vi "ErrorCheck.vi"(0 "Calib Baud rate":u32=9600, 1 "External VRN (COM8)":refnum<visa-resource-name>="COM8", 2 "Input Baud rate":u32=38400, 3 "TCS C VRN (COM4)":refnum<visa-resource-name>="COM4", 4 "TCS Contrôle Baud rate":u32=57600, 5 "TCS R VRN (COM7)":refnum<visa-resource-name>="COM7", 6 "TCS Requête Baud rate":u32=57600, 7 "MC bonOMM (COM3)":refnum<visa-resource-name>="COM3", 8 "Calib VRN (COM5)":refnum<visa-resource-name>="COM5", 9 "PathArray":path[](array[path])=[path "C:/UdeM/BonOMM-10/BonOMM-10_nocmd.vi", path "C:/UdeM/BonOMM-10/tracklogfiles", path "C:/UdeM/BonOMM-10/systemlogfiles", path "C:/UdeM/BonOMM-10/objectlibrary"], 10 "Table Baud rate":u32=38400, 12 "Table VRN (COM9)":refnum<visa-resource-name>="COM9") -> (11 "sortie librarypath":path=path "C:/UdeM/BonOMM-10/objectlibrary", 13 "sortie track":path=path "C:/UdeM/BonOMM-10/tracklogfiles", 14 "Table VRN OUT":refnum<visa-resource-name>="-1", 15 "sortie systemlog":path=path "C:/UdeM/BonOMM-10/systemlogfiles", 16 "Table Baud rate":u32=38400, 17 "Initialistion ok!":bool=TRUE, 18 "Calib VRN OUT":refnum<visa-resource-name>="COM5", 19 "MODE ?":i16=4, 20 "Calib Baud rate 2":u32=9600, 21 "External VRN OUT":refnum<visa-resource-name>="COM8", 22 "Input Baud rate 2":u32=38400, 23 "TCS C VRN OUT":refnum<visa-resource-name>="-1", 24 "TCS Contrôle Baud rate 2":u32=57600, 25 "TCS R VRN OUT":refnum<visa-resource-name>="-1", 26 "TCS Requête Baud rate":u32=57600, 27 "MC bonOMM OUT":refnum<visa-resource-name>="COM3")   [LabVIEW 2010]
uses:
  Comm/InitSerialPort_option.vi
panel:
  in  "search_MCB":bool
  in  "objectlibrarypath":path=path "C:/UdeM/BonOMM-10/objectlibrary" caption="Chemin du dossier des librairies"
  out "progress":i32(slide) min=0 max=100 step=5 scale=0.0..100.0
  out "MC Baud rate 2":u32=9600
  out "sortie vipath":path=path "C:/UdeM/BonOMM-10/BonOMM-10_nocmd.vi"
  in  "systemlogfilepath":path=path "C:/UdeM/BonOMM-10/systemlogfiles"
  in  "trackfilepath":path=path "C:/UdeM/BonOMM-10/tracklogfiles"
  in  "vipath":path=path "C:/UdeM/BonOMM-10/BonOMM-10_nocmd.vi"
  out "SPECTRO VRN OUT":refnum<visa-resource-name>="COM7"
  out "SPECTRO Baud rate":u32=57600
  out "ok 6":bool
  in  "MC Baud rate":u32=9600
  out "ok 5":bool
  out "ok 4":bool
  out "ok 3":bool
  out "ok 2":bool
  out "ok 1":bool
  in  "Annuler":bool
  in  "Démarrer":bool
  # "Chemin de l'application"
  # "Chemin des trackfiles"
  # "Chemin du dossier des logs système"
  # "Appuyer sur DÉMARRER lorsque vous\nêtes prêt à éxécuter BonOMM"
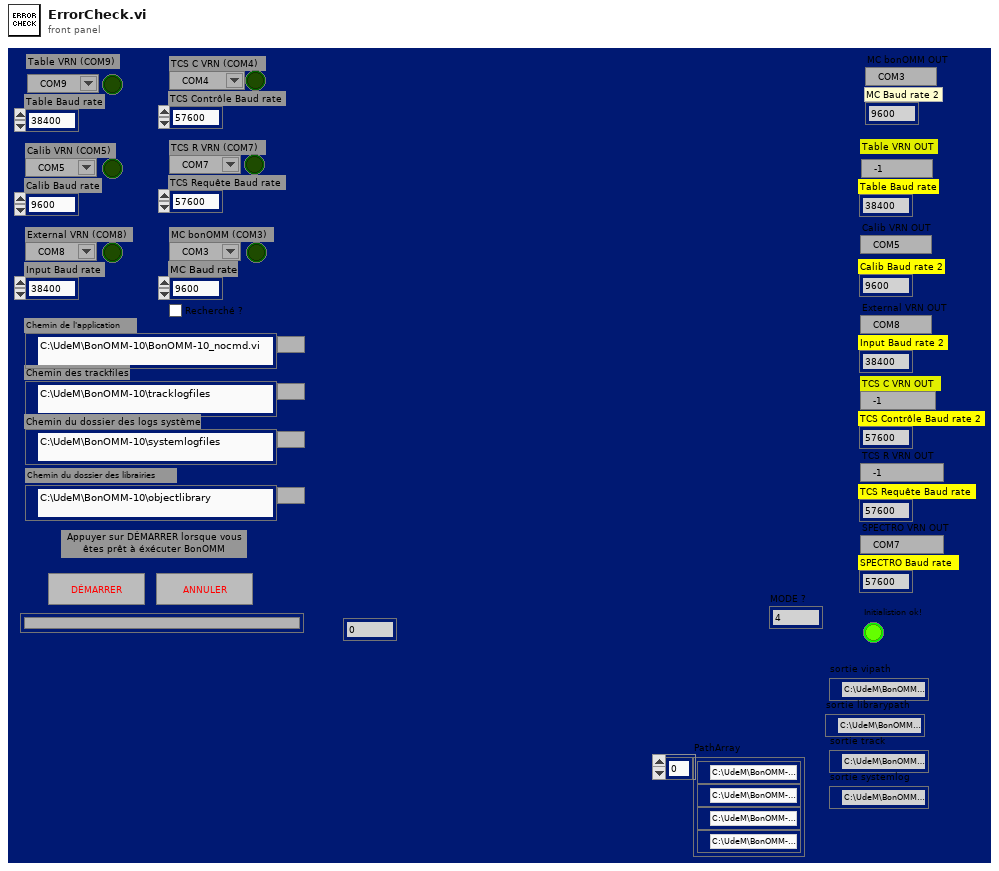
[diagram p1: front panel]
types:
  T1 = enum16{"Left Button", "Center Button", "Right Button", "Window Close"}
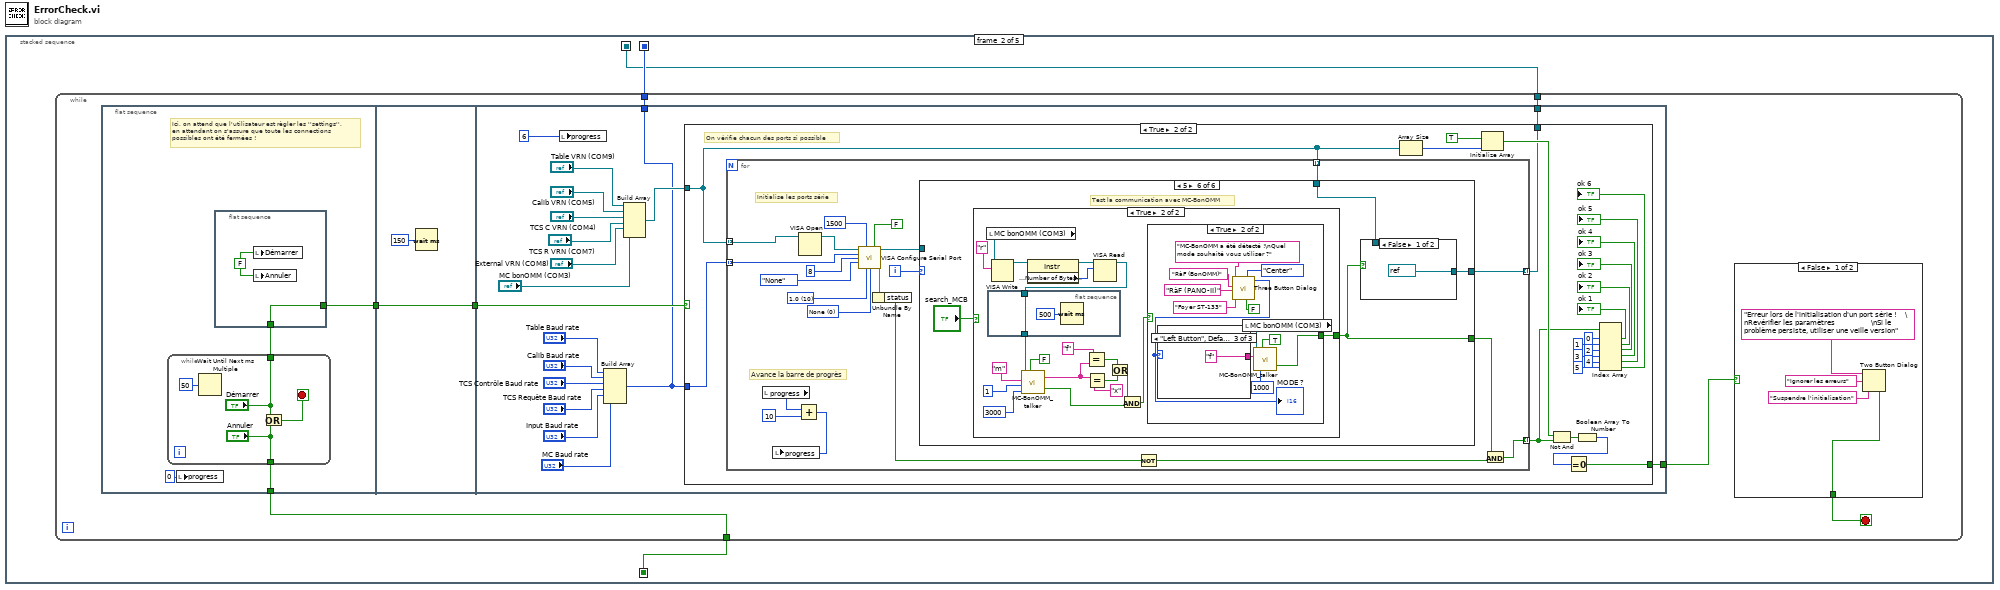
[diagram p0: block diagram]
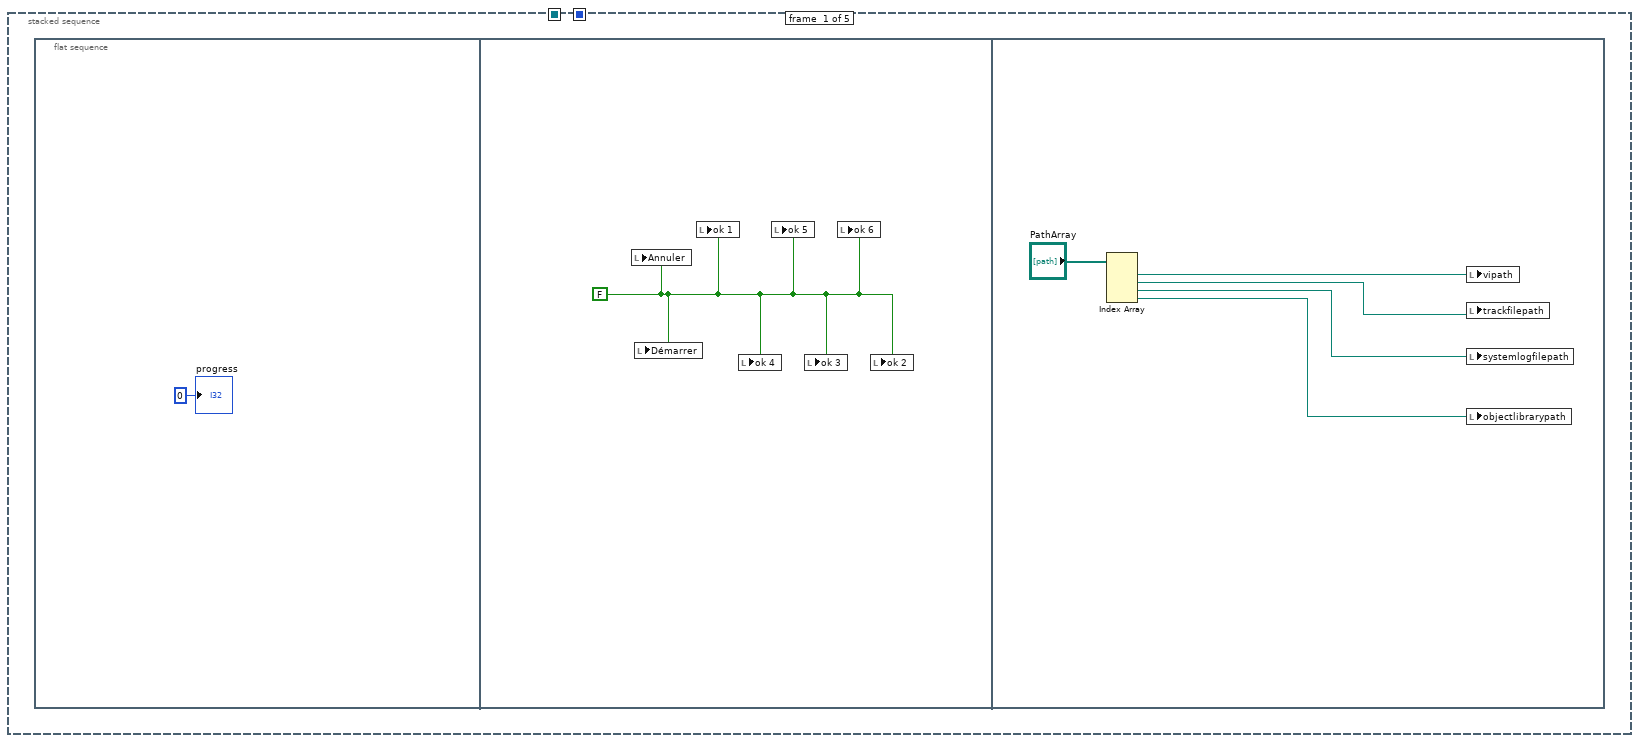
[diagram p2: hidden frame]
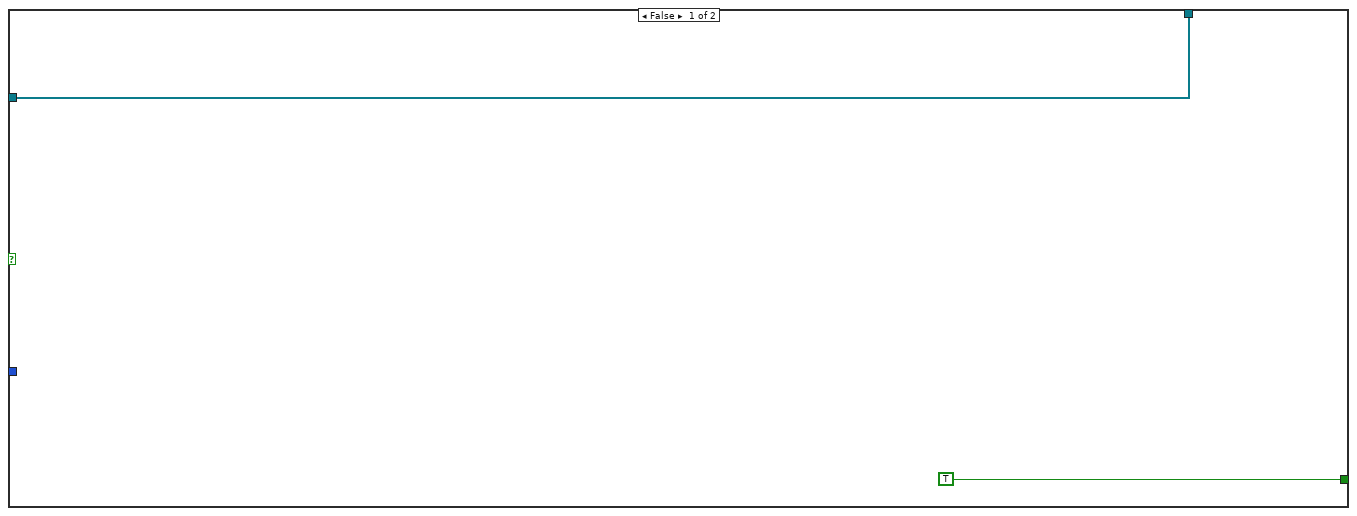
[diagram p4: hidden frame]
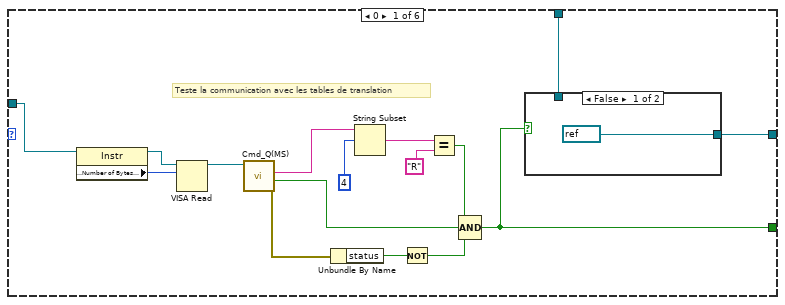
[diagram p5: hidden frame]
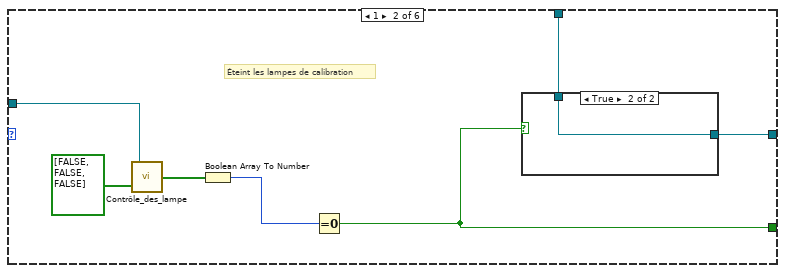
[diagram p7: hidden frame]
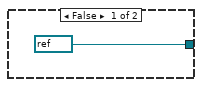
[diagram p8: hidden frame]
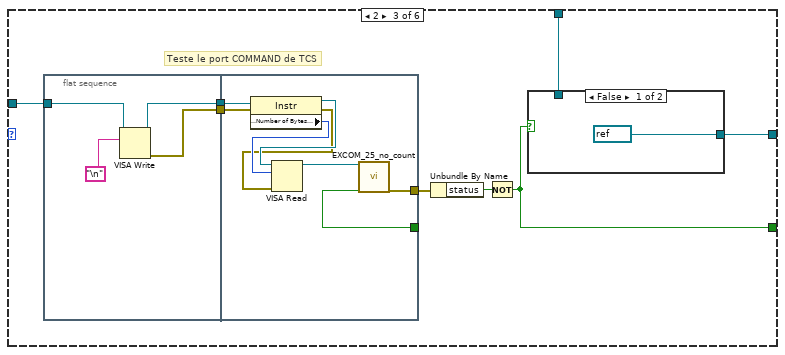
[diagram p9: hidden frame]
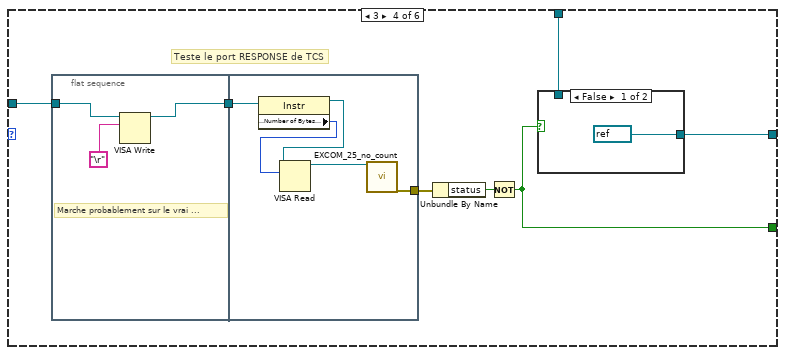
[diagram p11: hidden frame]
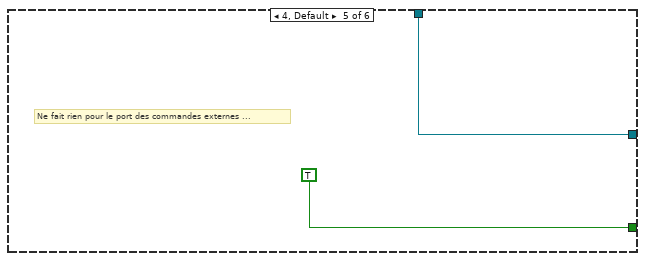
[diagram p13: hidden frame]
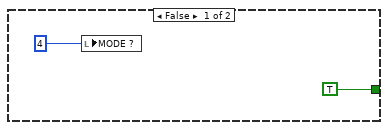
[diagram p15: hidden frame]
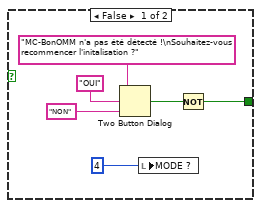
[diagram p16: hidden frame]
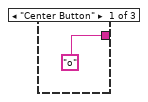
[diagram p17: hidden frame]
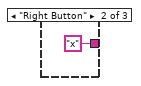
[diagram p18: hidden frame]
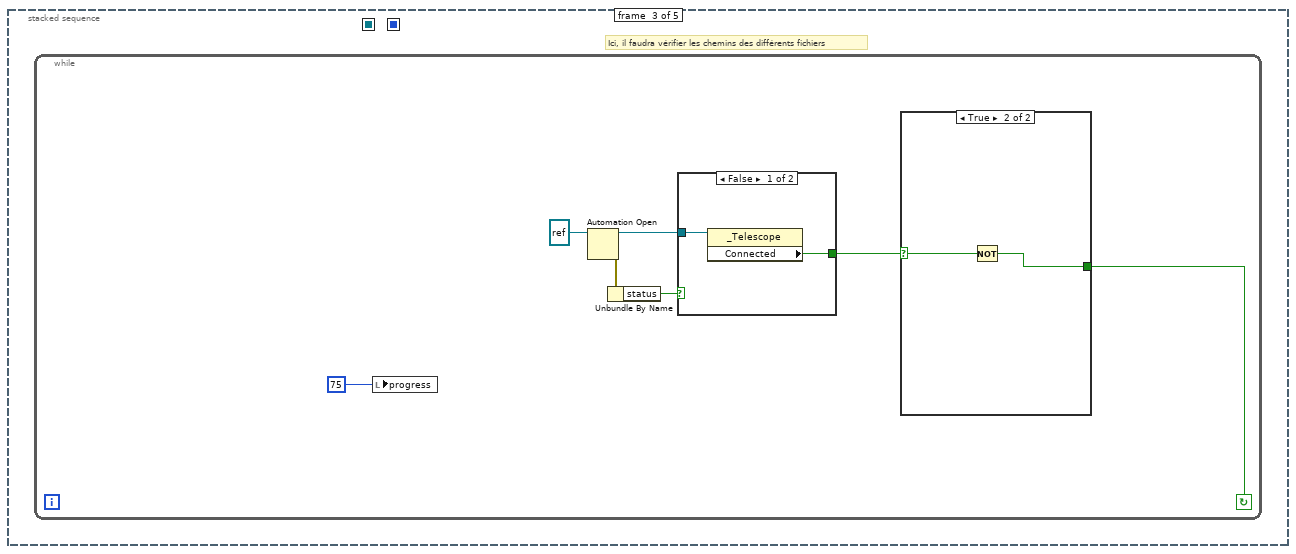
[diagram p19: hidden frame]
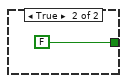
[diagram p20: hidden frame]
diagram:
  n1 = stacked-sequence {
    seq-local: [_ w10 _ _ _] -> [_ _ _ w238 _]
    seq-local: [_ w8 _ _ _] -> [_ _ _ w235 _]
    seq-local: [_ w9 _ _ _] -> [_ _ _ w234 _]
    frame #0 {
      n2 = flat-sequence {
        frame #0 {
          "progress" <- u8 0 ("progress")
        }
        frame #1 {
          w2 = FALSE
          n3 = local write "Annuler"(w2) -> ()
          n4 = local write "Démarrer"(w2) -> ()
          n5 = local write "ok 1"(w2) -> ()
          n6 = local write "ok 4"(w2) -> ()
          n7 = local write "ok 5"(w2) -> ()
          n8 = local write "ok 3"(w2) -> ()
          n9 = local write "ok 6"(w2) -> ()
          n10 = local write "ok 2"(w2) -> ()
        }
        frame #2 {
          n11 = Index Array(array="PathArray") -> (element #1=w6:path, element #2=w5:path, element #3=w4:path, element #4=w3:path)  [unwired: 4 in]
          n12 = local write "vipath"(w6) -> ()
          n13 = local write "trackfilepath"(w5) -> ()
          n14 = local write "systemlogfilepath"(w4) -> ()
          n15 = local write "objectlibrarypath"(w3) -> ()
        }
      }
    }
    frame #1 {
      n16 = while {
        tunnel: [w17] -> w10
        tunnel: [w14] -> w8
        tunnel: [w13] -> w9
        stop <- w15 stop-if-true
        n17 = flat-sequence {
          tunnel: [w26] -> w17
          tunnel: [w23] -> w12
          tunnel: w12 -> [w34]
          tunnel: [w34] -> w11
          tunnel: w11 -> [w52]
          tunnel: [w51] -> w16
          tunnel: [w36] -> w14
          tunnel: [w35] -> w13
          frame #0 {
            # "Ici, on attend que l'utilisateur est règler les ''settings'',\nen attendant on s'assure que toute les connections \npossibles ont été fermées !"
            n18 = while {
              tunnel: ["Annuler"] -> w26
              tunnel: ["Démarrer"] -> w24
              stop <- w32 stop-if-true
              n19 = Wait Until Next ms Multiple(millisecond multiple=u32 50) -> ()  [unwired: 1 out]
              n20 = Or(x="Démarrer", y="Annuler") -> (x .or. y?=w32:bool)
            }
            n21 = local write "progress"(0 ("progress")) -> ()
            n22 = flat-sequence {
              tunnel: [w28] -> w23
              tunnel: w24 -> [w28]
              frame #0 {
                w27 = FALSE ("Enable Termination\nChar (T)")
                n23 = local write "Démarrer"(w27) -> ()
                n24 = local write "Annuler"(w27) -> ()
              }
            }
          }
          frame #1 {
            n25 = Wait (ms)(milliseconds to wait=u32 150) -> ()  [unwired: 1 out]
          }
          frame #2 {
            n26 = local write "progress"(6 ("progress")) -> ()
            n27 = Build Array("Table Baud rate", "Calib Baud rate", "TCS Contrôle Baud rate", "TCS Requête Baud rate", "Input Baud rate", "MC Baud rate") -> (w35:u32[])
            n28 = Build Array("Table VRN (COM9)", "Calib VRN (COM5)", "TCS C VRN (COM4)", "TCS R VRN (COM7)", "External VRN (COM8)", "MC bonOMM (COM3)") -> (w38:refnum<visa-resource-name>[])
            n29 = case shown="True" w52 {
              tunnel: [TRUE w58] -> w51
              tunnel: w38 -> [w53 w56]
              tunnel: w35 -> [_ w57]
              tunnel: [w53 w55] -> w36
              frame False {
              }
              frame True {
                # "On vérifie chacun des ports si possible"
                n30 = for {
                  tunnel: w56 -> [w89] mode=indexing
                  tunnel: w57 -> [w97] mode=indexing
                  tunnel: [w79] -> w61 mode=indexing
                  tunnel: w56 -> [w78] mode=indexing
                  tunnel: [w77] -> w55 mode=indexing
                  i -> [w92]
                  w80 = u16 0 items=["None", "XON/XOFF", "RTS/CTS", "XON/XOFF & RTS/CTS", "DTR/DSR", "XON/XOFF & DTR/DSR"] ("flow control (0:none)")
                  w81 = u16 10 items=["1.0"=10, "1.5"=15, "2.0"=20] ("stop bits (10: 1 bit)")
                  # "Initialise les ports série"
                  # "Avance la barre de progrès"
                  n31 = local read "progress"() -> (w87:i32)
                  n32 = Add(x=w87, y=10) -> (x+y=w85:i32)
                  n33 = local write "progress"(w85) -> ()
                  n34 = VISA Open(VISA resource name=w89) -> (VISA resource name=w88:refnum<visa-resource-name>)  [unwired: 4 in, 1 out]
                  n35 = call-poly "VISA Configure Serial Port"("VISA resource name"=w88, "timeout (10sec)"=u32 1500, "Enable Termination\nChar (T)"=FALSE ("Enable Termination\nChar (T)"), "baud rate (9600)"=w97, "data bits (8)"=u16 8, "parity (0:none)"=enum16{"None", "Odd", "Even", "Mark", "Space"}."None", "stop bits (10: 1 bit)"=w81, "flow control (0:none)"=w80) -> ("VISA resource name out"=w95:refnum<visa-resource-name>, "error out"=w96:errorcluster)  [unwired: 6 in]
                  n36 = Unbundle By Name(w96) -> ("status"=w94:bool)
                  n37 = case shown="5" w92 {
                    tunnel: w95 -> [w113 w121 w132 w153 _ _]
                    tunnel: [w112 w118 w125 w147 TRUE ("Enable Termination\nChar (T)") w166] -> w93
                    tunnel: w78 -> [w110 w116 w129 w150 w164 w167]
                    tunnel: [w111 w117 w128 w151 w164 w168] -> w77
                    frame 0 {
                      # "Teste la communication avec les tables de translation"
                      n38 = property class="Instr"(reference=w113) -> (reference out=w109:refnum<visa-resource-name>, "Serial Settings:Number of Bytes at Serial Port"=w108:u32)  [unwired: 1 in, 1 out]
                      n39 = VISA Read(VISA resource name=w109, byte count=w108) -> (VISA resource name out=w107:refnum<visa-resource-name>)  [unwired: 1 in, 3 out]
                      n40 = call "Cmd_Q(MS).vi"("VISA resource name IN"=w107) -> ("error out"=w99:errorcluster, "OK Done"=w101:bool, "Q String"=w104:string)  [unwired: 3 in, 5 out]
                      n41 = Unbundle By Name(w99) -> ("status"=w100:bool)
                      n42 = String Subset(string=w104, offset (0)=4) -> (substring=w103:string)  [unwired: 1 in]
                      n43 = Not(x=w100) -> (.not. x?=w98:bool)
                      n44 = Equal?(x=w103, y="R") -> (x = y?=w105:bool)
                      n45 = Compound Arithmetic op=AND(w105, w101, w98) -> (w112:bool)
                      n46 = case shown="False" w112 {
                        tunnel: [refnum<visa-resource-name> "-1" ("Table VRN") w115] -> w111
                        tunnel: w110 -> [_ w115]
                        frame False {
                        }
                        frame True {
                        }
                      }
                    }
                    frame 1 {
                      # "Éteint les lampes de calibration"
                      n47 = call "Contrôle_des_lampe.vi"("VISA resource name"=w121, "Status In"=bool[] [FALSE, FALSE, FALSE]) -> ("Status Out"=w120:bool[])  [unwired: 2 out]
                      n48 = Boolean Array To Number(Boolean array=w120) -> (number=w119:u32)
                      n49 = Equal To 0?(x=w119) -> (x = 0?=w118:bool)
                      n50 = case shown="True" w118 {
                        tunnel: [refnum<visa-resource-name> "-1" ("Table VRN") w124] -> w117
                        tunnel: w116 -> [_ w124]
                        frame False {
                        }
                        frame True {
                        }
                      }
                    }
                    frame 2 {
                      # "Teste le port COMMAND de TCS"
                      n51 = flat-sequence {
                        tunnel: w132 -> [w138]
                        tunnel: [w137] -> w131
                        tunnel: [w135] -> w130
                        tunnel: [w146] -> _
                        tunnel: w131 -> [w143]
                        tunnel: w130 -> [w141]
                        tunnel: [w139] -> w126
                        frame #0 {
                          n52 = VISA Write(VISA resource name=w138, write buffer="\n") -> (VISA resource name out=w137:refnum<visa-resource-name>, error out=w135:errorcluster)  [unwired: 1 in, 1 out]
                        }
                        frame #1 {
                          n53 = property class="Instr"(reference=w143, error in=w141) -> (reference out=w145:refnum<visa-resource-name>, error out=w140:errorcluster, "Serial Settings:Number of Bytes at Serial Port"=w144:u32)
                          n54 = VISA Read(VISA resource name=w145, byte count=w144, error in (no error)=w140) -> (VISA resource name out=w142:refnum<visa-resource-name>)  [unwired: 3 out]
                          n55 = call "EXCOM_25_no_count.vi"("VISA resource name"=w142) -> ("OK Done"=w146:bool, "error out"=w139:errorcluster)  [unwired: 4 in, 13 out]
                        }
                      }
                      n56 = Unbundle By Name(w126) -> ("status"=w127:bool)
                      n57 = Not(x=w127) -> (.not. x?=w125:bool)
                      n58 = case shown="False" w125 {
                        tunnel: w129 -> [_ w134]
                        tunnel: [refnum<visa-resource-name> "-1" ("Table VRN") w134] -> w128
                        frame False {
                        }
                        frame True {
                        }
                      }
                    }
                    frame 3 {
                      # "Teste le port RESPONSE de TCS"
                      n59 = flat-sequence {
                        tunnel: w153 -> [w158]
                        tunnel: [w157] -> w152
                        tunnel: w152 -> [w161]
                        tunnel: [w159] -> w149
                        frame #0 {
                          # "Marche probablement sur le vrai ..."
                          n60 = VISA Write(VISA resource name=w158, write buffer="\r") -> (VISA resource name out=w157:refnum<visa-resource-name>)  [unwired: 1 in, 2 out]
                        }
                        frame #1 {
                          n61 = property class="Instr"(reference=w161) -> (reference out=w163:refnum<visa-resource-name>, "Serial Settings:Number of Bytes at Serial Port"=w162:u32)  [unwired: 1 in, 1 out]
                          n62 = VISA Read(VISA resource name=w163, byte count=w162) -> (VISA resource name out=w160:refnum<visa-resource-name>)  [unwired: 1 in, 3 out]
                          n63 = call "EXCOM_25_no_count.vi"("VISA resource name"=w160) -> ("error out"=w159:errorcluster)  [unwired: 4 in, 14 out]
                        }
                      }
                      n64 = Unbundle By Name(w149) -> ("status"=w148:bool)
                      n65 = Not(x=w148) -> (.not. x?=w147:bool)
                      n66 = case shown="False" w147 {
                        tunnel: w150 -> [_ w155]
                        tunnel: [refnum<visa-resource-name> "-1" ("Table VRN") w155] -> w151
                        frame False {
                        }
                        frame True {
                        }
                      }
                    }
                    frame 4, Default {
                      # "Ne fait rien pour le port des commandes externes ..."
                    }
                    frame 5 {
                      # "Test la communication avec MC-BonOMM"
                      n67 = case shown="True" "search_MCB" {
                        tunnel: [TRUE ("ok ?") w176] -> w166
                        frame False {
                          n68 = local write "MODE ?"(i16 4 ("MODE ?")) -> ()
                        }
                        frame True {
                          n69 = local read "MC bonOMM (COM3)"() -> (w192:refnum<visa-resource-name>)
                          n70 = flat-sequence {
                            tunnel: w175 -> [w195]
                            tunnel: [w195] -> w174
                            frame #0 {
                              n71 = Wait (ms)(milliseconds to wait=u32 500) -> ()  [unwired: 1 out]
                            }
                          }
                          n72 = VISA Write(VISA resource name=w192, write buffer="r" ("Commande")) -> (VISA resource name out=w191:refnum<visa-resource-name>)  [unwired: 1 in, 2 out]
                          n73 = call "MC-BonOMM_talker.vi"("MC-BonOMM VRN"=w174, "Commande"="m", "byte count"=u32 1, "Timeout (ms)"=3000, "answer=command?"=FALSE) -> ("Answer"=w178:string, "ok ?"=w179:bool)
                          n74 = property class="Instr"(reference=w191) -> (reference out=w190:refnum<visa-resource-name>, "Serial Settings:Number of Bytes at Serial Port"=w189:u32)  [unwired: 1 in, 1 out]
                          n75 = Equal?(x="f", y=w178) -> (x = y?=w183:bool)
                          n76 = Equal?(x=w178, y="x") -> (x = y?=w184:bool)
                          n77 = VISA Read(VISA resource name=w190, byte count=w189) -> (VISA resource name out=w175:refnum<visa-resource-name>)  [unwired: 1 in, 3 out]
                          n78 = Or(x=w183, y=w184) -> (x .or. y?=w180:bool)
                          n79 = And(x=w180, y=w179) -> (x .and. y?=w177:bool)
                          n80 = case shown="True" w177 {
                            tunnel: [w197 w211] -> w176
                            frame False {
                              n81 = Two Button Dialog(message="MC-BonOMM n'a pas été détecté !\nSouhaitez-vous recommencer l'initalisation ?", 1:"NON" ("F button name (\"Cancel\")"), 2:"OUI" ("T button name (\"OK\")")) -> (T button?=w198:bool)
                              n82 = local write "MODE ?"(i16 4 ("MODE ?")) -> ()
                              n83 = Not(x=w198) -> (.not. x?=w197:bool)
                            }
                            frame True {
                              n84 = call <vilib>:"Three Button Dialog.vi"("Allow user to close window? (TRUE)"=FALSE, "Justify Message (Left)"=enum16{"Left", "Center", "Right"}."Center", "Right Button Text (\"Cancel\")"="Foyer ST-133" ("F button name (\"Cancel\")"), "Center Button Text (\"No\")"="RàF (PANO-II)" ("F button name (\"Cancel\")"), "Left Button Text (\"Yes\")"="RàF (BonOMM)" ("T button name (\"OK\")"), "message"="MC-BonOMM a été détecté !\nQuel mode souhaité vous utiliser ?") -> ("Which Button?"=w203:T1)  [unwired: 5 in]
                              "MODE ?" <- w203
                              n85 = case shown="\"Left Button\", Default" w203 {
                                tunnel: ["o" "x" "f"] -> w202
                                frame "Center Button" {
                                }
                                frame "Right Button" {
                                }
                                frame "Left Button", Default {
                                }
                              }
                              n86 = local read "MC bonOMM (COM3)"() -> (w210:refnum<visa-resource-name>)
                              n87 = call "MC-BonOMM_talker.vi"("MC-BonOMM VRN"=w210, "Commande"=w202, "Timeout (ms)"=1000, "answer=command?"=TRUE) -> ("ok ?"=w211:bool)  [unwired: 1 in, 1 out]
                            }
                          }
                        }
                      }
                      n88 = case shown="False" w166 {
                        tunnel: w167 -> [_ w171]
                        tunnel: [refnum<visa-resource-name> "-1" ("Table VRN") w171] -> w168
                        frame False {
                        }
                        frame True {
                        }
                      }
                    }
                  }
                  n89 = Not(x=w94) -> (.not. x?=w91:bool)
                  n90 = And(x=w93, y=w91) -> (x .and. y?=w79:bool)
                }
                n91 = Array Size(array=w56) -> (size(s)=w76:i32)
                n92 = Initialize Array(TRUE ("Enable Termination\nChar (T)"), w76) -> (w74:bool[])
                n93 = Not And(1:w61, 2:w74) -> (0:w73:bool[])
                n94 = Boolean Array To Number(Boolean array=w73) -> (number=w72:u32)
                n95 = Equal To 0?(x=w72) -> (x = 0?=w58:bool)
                n96 = Index Array(array=w61, index #1=0 ("index"), index #2=1 ("index"), index #3=2 ("index"), index #4=3 ("index"), index #5=4 ("index"), index #6=5 ("index")) -> (element #1=→"ok 1":bool, element #2=→"ok 2":bool, element #3=→"ok 3":bool, element #4=→"ok 4":bool, element #5=→"ok 5":bool, element #6=→"ok 6":bool)
              }
            }
          }
        }
        n97 = case shown="False" w16 {
          selector: w16 -> [_ w22]
          tunnel: [w18 w22] -> w15
          frame False {
            n98 = Two Button Dialog(message="Erreur lors de l'initialisation d'un port série !    \nRevérifier les paramètres                  \nSi le problème persiste, utiliser une veille version", 1:"Suspendre l'initialisation" ("F button name (\"Cancel\")"), 2:"Ignorer les erreurs" ("T button name (\"OK\")")) -> (T button?=w18:bool)
          }
          frame True {
          }
        }
      }
    }
    frame #2 {
      # "Ici, il faudra vérifier les chemins des différents fichiers"
      n99 = while {
        stop <- w223 continue-if-true
        n100 = local write "progress"(75 ("progress")) -> ()
        n101 = Automation Open(Automation Refnum=refnum<k7> refnum ("reference")) -> (Automation Refnum=w218:refnum<k7>, error out=w217:errorcluster)  [unwired: 3 in]
        n102 = Unbundle By Name(w217) -> ("status"=w220:bool)
        n103 = case shown="False" w220 {
          tunnel: w218 -> [w225 _]
          tunnel: [w224 FALSE ("Connected")] -> w221
          frame False {
            n104 = property class="_Telescope"(reference=w225) -> ("Connected"=w224:bool)  [unwired: 1 in, 2 out]
          }
          frame True {
          }
        }
        n105 = case shown="True" w221 {
          selector: w221 -> [_ w232]
          tunnel: [w227 w231] -> w223
          frame False {
            n106 = Two Button Dialog(message=" Problème avec StarryNight ou\navec le simulateur de télescope\nAssurez-vous que le simulateur\n  de télescope est connecté !", 1:"Ignorer l'erreur" ("F button name (\"Cancel\")"), 2:"Réessayer" ("T button name (\"OK\")")) -> (T button?=w227:bool)
          }
          frame True {
            n107 = Not(x=w232) -> (.not. x?=w231:bool)
          }
        }
      }
    }
    frame #3 {
      n108 = Not(x=w238) -> (.not. x?=→"Initialistion ok!":bool)
      n109 = case shown="False" w238 {
        tunnel: w234 -> [w260 _]
        tunnel: w235 -> [w247 w271]
        tunnel: [w247 w271] -> w237
        frame False {
          n110 = Index Array(array=w260, index #1=0 ("index"), index #2=1 ("index"), index #3=2 ("index"), index #4=3 ("index"), index #5=4 ("index"), index #6=5 ("index")) -> (element #1=→"Table Baud rate":u32, element #2=→"Calib Baud rate 2":u32, element #3=→"TCS Contrôle Baud rate 2":u32, element #4=→"TCS Requête Baud rate":u32, element #5=→"Input Baud rate 2":u32, element #6=→"MC Baud rate 2":u32)
          n111 = Index Array(array=w247, index #1=0 ("index"), index #2=1 ("index"), index #3=2 ("index"), index #4=3 ("index"), index #5=4 ("index"), index #6=5 ("index")) -> (element #1=→"Table VRN OUT":refnum<visa-resource-name>, element #2=→"Calib VRN OUT":refnum<visa-resource-name>, element #3=→"TCS C VRN OUT":refnum<visa-resource-name>, element #4=→"TCS R VRN OUT":refnum<visa-resource-name>, element #5=→"External VRN OUT":refnum<visa-resource-name>, element #6=→"MC bonOMM OUT":refnum<visa-resource-name>)
        }
        frame True {
          n112 = One Button Dialog(message="Erreur lors de l'initialisation") -> ()  [unwired: 1 in, 1 out]
        }
      }
      n113 = local write "progress"(90 ("progress")) -> ()
      n114 = for {
        tunnel: w237 -> [w244] mode=indexing
        i -> [w243]
        n115 = Multiply(x=2, y=w243) -> (x*y=w242:i32)
        n116 = VISA Close(VISA resource name=w244) -> ()  [unwired: 1 in, 1 out]
        n117 = Add(x=w242, y=90 ("progress")) -> (x+y=w239:i32)
        n118 = local write "progress"(w239) -> ()
      }
    }
    frame #4 {
      "sortie systemlog" <- "systemlogfilepath"
      "sortie vipath" <- "vipath"
      "sortie track" <- "trackfilepath"
      "sortie librarypath" <- "objectlibrarypath"
    }
  }
